vi "onStop.vi"(8 "error in (no error)":errorcluster, 11 "Inst.Transport":refnum<class "Inst.Transport.lvclass">) -> (0 "error out":errorcluster, 3 "Inst.Transport out":refnum<class "Inst.Transport.lvclass">)   [LabVIEW 2019, in "Inst.Transport.lvclass"]
uses:
  Inst.Transport.lvclass
  Inst.Transport.lvclass/Inst.Transport.ctl
  <userlib>/LevyLab/Instrument Framework/Instrument Types/SCPI/Instrument.SCPI.lvclass
panel:
  # "For instructions on how to use the JKI State Machine Objects, examples and video tutorials, visit:\nhttp://jki.net/state-machine-objects/\n\nJKI State Machine Objects™\nhttp://jki.net/state-machine-objects/\nCopyright (C) 2005-2015, JKI <info@jki.net>\nALL RIGHTS RESERVED"
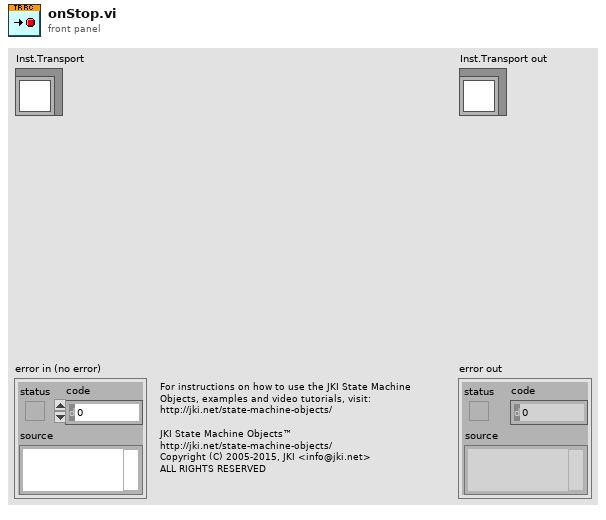
[diagram p1: front panel]
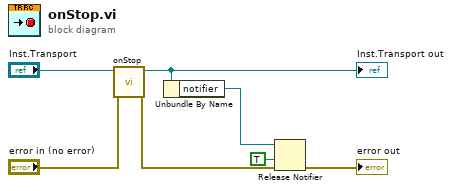
[diagram p0: block diagram]
diagram:
  n1 = call-parent "onStop.vi"("error in (no error)"="error in (no error)", "SMO"="Inst.Transport") -> ("error out"=w2:errorcluster, "SMO out"=w6:refnum<class "Inst.Transport.lvclass">)  [unwired: 8 in]
  "Inst.Transport out" <- w6
  n2 = Unbundle By Name(w6) -> ("notifier"=w5:refnum<notifier>)
  n3 = Release Notifier(notifier=w5, force destroy? (F)=TRUE, error in (no error)=w2) -> (error out=→"error out":errorcluster)  [unwired: 2 out]
